vi "Tank Drive.vi"(6 "Drive Dev Ref":T1[](array[typedef]), 7 "Swerve Dev Ref":T1[](array[typedef]), 8 "error in":errorcluster, 10 "Right Axis":dbl format="%#_13g", 11 "Left Axis":dbl format="%#_13g") -> (0 "error out":errorcluster)   [LabVIEW 2016, in "Huskie Swerve.lvlib"]
uses:
  Huskie Swerve.lvlib
  <vilib>/Rock Robotics/WPI/MotorControl/WPI_MotorControlDeviceRef.ctl
  <vilib>/Rock Robotics/WPI/MotorControl/WPI_MotorControlType.ctl
  <vilib>/Rock Robotics/SystemInterfaces/DIO/FPGA_DIOPWMChannel.ctl
  <vilib>/Rock Robotics/WPI/PWM/WPI_PWMDeadband.ctl
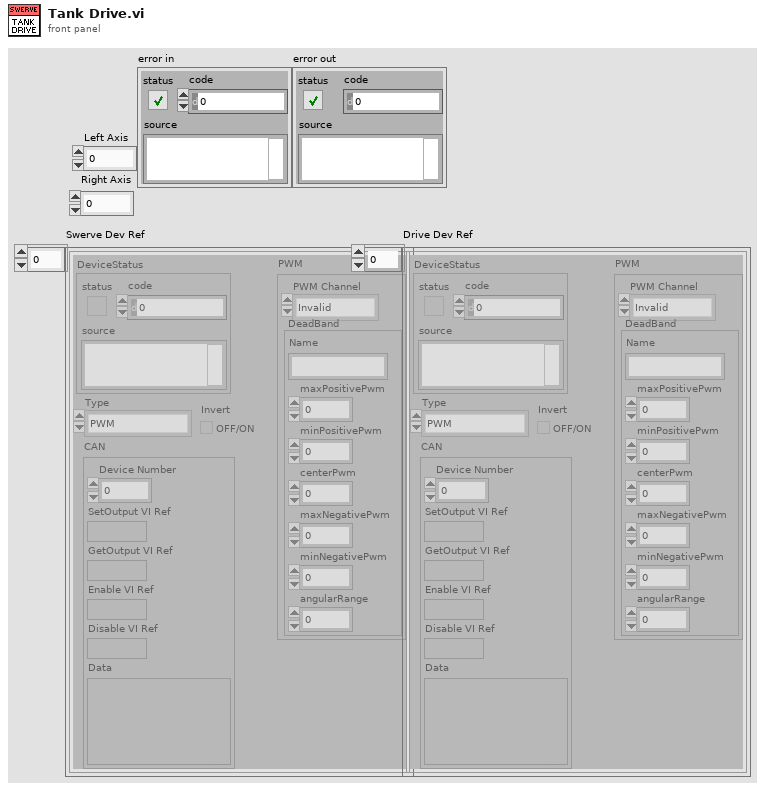
[diagram p1: front panel]
types:
  T1 = typedef "WPI_MotorControlDeviceRef.ctl" = cluster{"DeviceStatus":errorcluster, "Type":T2, "PWM":cluster{"PWM Channel":T3, "DeadBand":T4}, "CAN":cluster{"Device Number":u8, "SetOutput VI Ref":variant, "GetOutput VI Ref":variant, "Enable VI Ref":variant, "Disable VI Ref":variant, "Data":variant}, "Invert":bool}
  T2 = typedef "WPI_MotorControlType.ctl" = enum16{"PWM", "CAN"}
  T3 = typedef "FPGA_DIOPWMChannel.ctl" = enum8{"PWM 0", "PWM 1", "PWM 2", "PWM 3", "PWM 4", "PWM 5", "PWM 6", "PWM 7", "PWM 8", "PWM 9", "PWM MXP 0", "PWM MXP 1", "PWM MXP 2", "PWM MXP 3", "PWM MXP 4", "PWM MXP 5", "PWM MXP 6", "PWM MXP 7", "PWM MXP 8", "PWM MXP 9", "Invalid"}
  T4 = typedef "WPI_PWMDeadband.ctl" = cluster{"Name":string, "maxPositivePwm":i32, "minPositivePwm":i32, "centerPwm":i32, "maxNegativePwm":i32, "minNegativePwm":i32, "angularRange":u16}
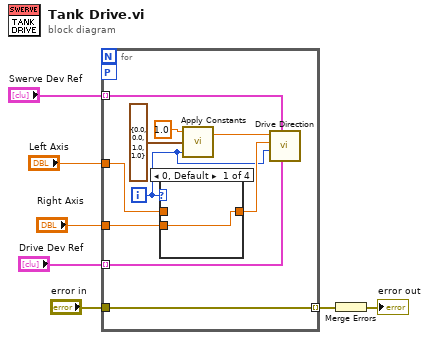
[diagram p0: block diagram]
diagram:
  n1 = for {
    workers-P: _ -> [_]
    tunnel: "Left Axis" -> [w14]
    tunnel: "Right Axis" -> [w13]
    tunnel: "Swerve Dev Ref" -> [w11] mode=indexing
    tunnel: "Drive Dev Ref" -> [w10] mode=indexing
    tunnel: [w9] -> w2 mode=indexing
    tunnel: "error in" -> [w9]
    i -> [w8]
    n2 = case shown="0, Default" w8 {
      tunnel: w14 -> [_ w19 w20 _]
      tunnel: w13 -> [w18 _ _ w21]
      tunnel: [w18 w19 w20 w21] -> w12
      frame 0, Default {
      }
      frame 1 {
      }
      frame 2 {
      }
      frame 3 {
      }
    }
    n3 = call "Apply Constants.vi"("Module Number"=w8, "constants cluster"=cluster{"a":dbl, "b":dbl, "c":dbl, "d":dbl} {"a"=0.0, "b"=0.0, "c"=1.0, "d"=1.0}, "Max Speed or 1"=1.0) -> ("Desired Direction (rad)"=w17:dbl)  [unwired: 1 out]
    n4 = call "Drive Direction.vi"("Drive Dev Ref"=w10, "Swerve Dev Ref"=w11, "Module Number"=w8, "Wheel Power"=w12, "Desired direction (radians)"=w17) -> ()  [unwired: 7 in]
  }
  n5 = Merge Errors(w2) -> (→"error out":errorcluster)
